vi "ScopeTraceFGV_5.vi"(9 "output cluster 2":T1, 10 "command":T2, 11 "Nr.":i32) -> (1 "output cluster 2":T1)   [LabVIEW 2013]
uses:
  scopeTrace_TupDef.ctl
  commandForScopeTrace.ctl
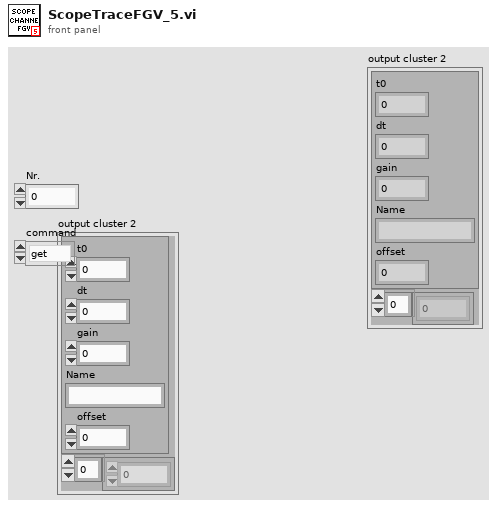
[diagram p1: front panel]
types:
  T1 = typedef "scopeTrace_TupDef.ctl" = cluster{cluster{"t0":dbl, "dt":dbl, "gain":dbl, "Name":string, "offset":dbl}, i16[]}
  T2 = typedef "commandForScopeTrace.ctl" = enum16{"get", "set", "init", "get ALL"}
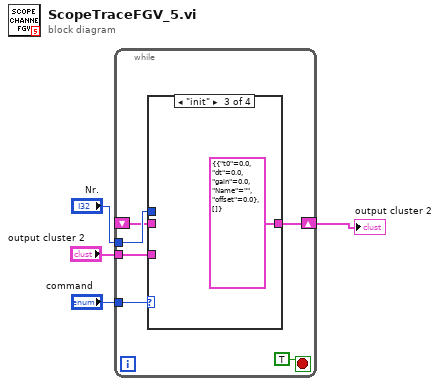
[diagram p0: block diagram]
diagram:
  n1 = while {
    shift-right: [w7] -> w1
    shift-left: _ -> [w5]
    tunnel: "Nr." -> [w9]
    tunnel: "output cluster 2" -> [w8]
    tunnel: "command" -> [w6]
    stop <- TRUE stop-if-true
    n2 = case shown="\"init\"" w6 {
      tunnel: w9 -> [_ _ _ _]
      tunnel: w8 -> [_ _ _ w14]
      tunnel: [w11 w12 T1 {{"t0"=0.0, "dt"=0.0, "gain"=0.0, "Name"="", "offset"=0.0}, []} ("output cluster 2") w14] -> w7
      tunnel: w5 -> [w11 w12 _ _]
      frame "get", Default {
      }
      frame "get ALL" {
      }
      frame "init" {
      }
      frame "set" {
      }
    }
  }
  "output cluster 2" <- w1
